vi "Modules Selector.vi"(7 "Scan All":bool, 8 "Module In Dependencies?":bool[](array[boolean]), 10 "Modules Types In":T1[](array[typedef]), 11 "DQMH Modules In":refnum<vi>[](array[refnum])) -> (0 "Module In Dependencies?Out":bool[](array[boolean]), 1 "Descriptions":string[](array[string]), 2 "Modules Types Out":T1[](array[typedef]), 3 "DQMH Modules Out":refnum<vi>[](array[refnum]), 4 "Scan?":bool)   [LabVIEW 2021, in "Panther Dashboard.lvlib"]
uses:
  Panther Dashboard.lvlib
  Module type--enum.ctl
  Module to scan--cluster.ctl
panel:
  in  "DQMH Modules found in Project":T2[](array[typedef])
  in  "Scan Selection":bool
  in  "Select/Unselect All":bool
types:
  T1 = typedef "Panther Dashboard.lvlib/Module type--enum.ctl" = enum16{"Module type: Singleton", "Module type: Cloneable"}
  T2 = typedef "Panther Dashboard.lvlib/Module to scan--cluster.ctl" = cluster{"Module Name":string, "Description":string, "Scan?":bool, "Dependency":bool}
  T3 = enum8{"Enabled", "Disabled", "Disabled and Grayed Out"}
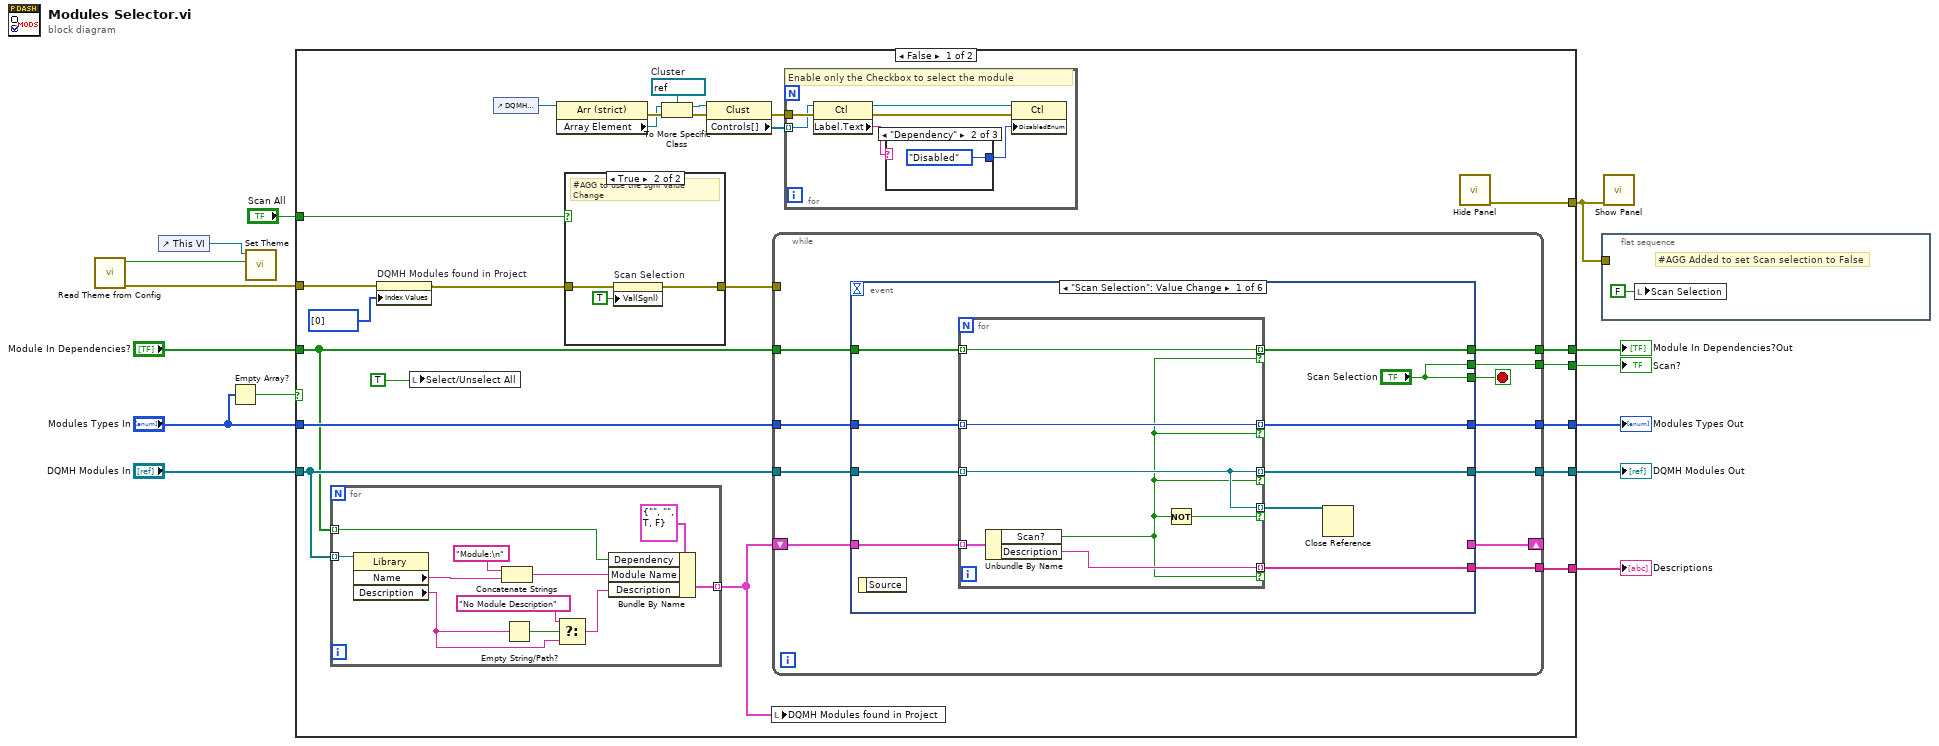
[diagram p0: block diagram]
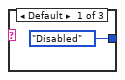
[diagram p3: hidden frame]
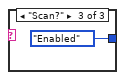
[diagram p4: hidden frame]
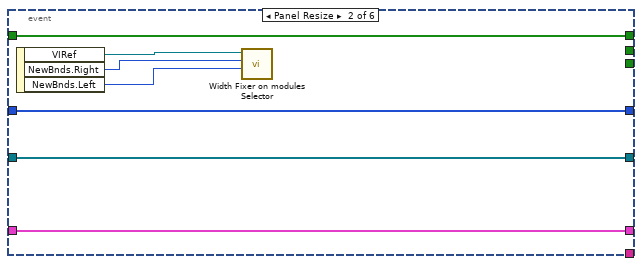
[diagram p5: hidden frame]
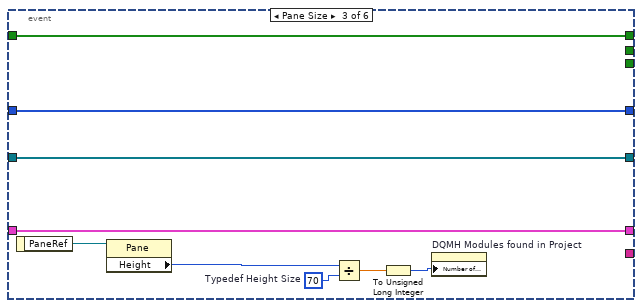
[diagram p6: hidden frame]
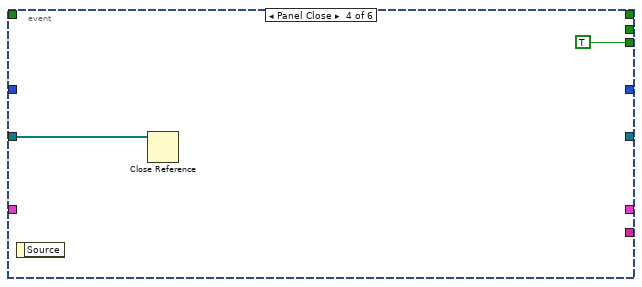
[diagram p7: hidden frame]
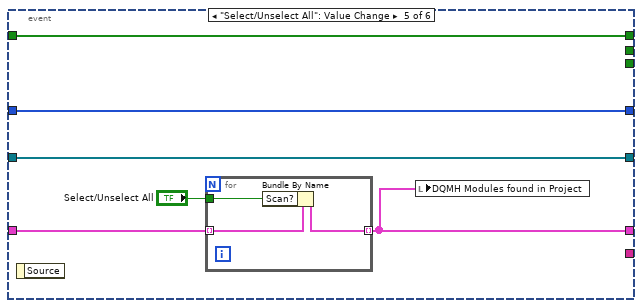
[diagram p8: hidden frame]
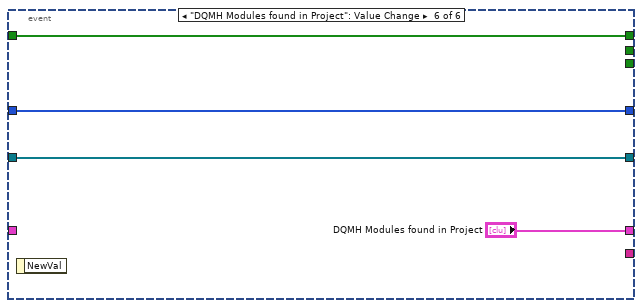
[diagram p9: hidden frame]
diagram:
  n1 = call "Read Theme from Config.vi"() -> ("error out"=w14:errorcluster, "Theme"=w9:bool)  [unwired: 10 in]
  n2 = control-ref of="This VI"() -> (w10:refnum<vi>)
  n3 = Empty Array?(array="Modules Types In") -> (empty?=w7:bool)
  n4 = call "Set Theme.vi"("Dark?"=w9, "VI in"=w10) -> ()  [unwired: 10 in]
  n5 = case shown="False" w7 {
    tunnel: "DQMH Modules In" -> [w29 _]
    tunnel: [w33 _] -> w6
    tunnel: "Modules Types In" -> [w32 _]
    tunnel: [w31 _] -> w12
    tunnel: [w30 _] -> w11
    tunnel: w14 -> [w37 _]
    tunnel: [w38 _] -> w2
    tunnel: "Module In Dependencies?" -> [w24 _]
    tunnel: [w25 _] -> w4
    tunnel: [w18 _] -> w3
    tunnel: "Scan All" -> [w15 _]
    frame False {
      w19 = refnum<vi> refnum  # Cluster
      n6 = for {
        tunnel: w29 -> [w62] mode=indexing
        tunnel: [w61] -> w28 mode=indexing
        tunnel: w24 -> [w52] mode=indexing
        n7 = property class="Library"(reference=w62) -> ("Name"=w59:string, "Description"=w57:string)  [unwired: 1 in, 2 out]
        n8 = Concatenate Strings("Module:\n" ("string"), w59) -> (w54:string)
        n9 = Empty String/Path?(string/path=w57) -> (empty?=w58:bool)
        n10 = Select(t="No Module Description", s=w58, f=w57) -> (s? t:f=w56:string)
        n11 = Bundle By Name(cluster=T2 {"Module Name"="", "Description"="", "Scan?"=TRUE, "Dependency"=FALSE} ("Module"), "Dependency"=w52, "Module Name"=w54, "Description"=w56) -> (w61:T2)
      }
      n12 = property on="DQMH Modules found in Project" class="Arr (strict)"(error in=w37, "Index Values"=u32[] [0]) -> (error out=w16:errorcluster)  [unwired: 1 in, 1 out]
      n13 = local write "Select/Unselect All"(TRUE ("Select /Unselect All Modules")) -> ()
      n14 = control-ref of="DQMH Modules found in Project"() -> (w20:refnum<vi>)
      n15 = property class="Arr (strict)"(reference=w20) -> (error out=w34:errorcluster, "Array Element"=w21:refnum<vi>)  [unwired: 1 in, 1 out]
      n16 = case shown="True" w15 {
        tunnel: [w39 w42] -> w17
        tunnel: w16 -> [w39 w41]
        frame False {
        }
        frame True {
          # "#AGG to use the sgnl Value Change"
          n17 = property on="Scan Selection" class="Bool (strict)"(error in=w41, "Val(Sgnl)"=TRUE ("Value (Signaling)")) -> (error out=w42:errorcluster)  [unwired: 1 in, 1 out]
        }
      }
      n18 = To More Specific Class(target class=w19, reference=w21, error in=w34) -> (specific class reference=w22:refnum<vi>, error out=w35:errorcluster)
      n19 = property class="Clust"(reference=w22, error in=w35) -> (error out=w36:errorcluster, "Controls[]"=w23:refnum<vi>[])  [unwired: 1 out]
      n20 = local write "DQMH Modules found in Project"(w28) -> ()
      n21 = while {
        shift-right: [w72] -> _
        shift-left: w28 -> [w73]
        tunnel: w29 -> [w71]
        tunnel: [w70] -> w33
        tunnel: w32 -> [w69]
        tunnel: [w68] -> w31
        tunnel: [w67] -> w30
        tunnel: w24 -> [w66]
        tunnel: [w65] -> w25
        tunnel: [w63] -> w18
        tunnel: w17 -> [_]
        stop <- w64 stop-if-true
        n22 = event shown="[0] \"Scan Selection\": Value Change" {
          selector: _ -> [_ _ _ _ _ _]
          dyn-events: _ -> [_ _ _ _ _ _]
          timeout: _ -> [_ _ _ _ _ _]
          tunnel: w73 -> [w83 w95 w102 _ w112 _]
          tunnel: ["Scan Selection" _ _ TRUE ("All") _ _] -> w64
          tunnel: [_ w95 w102 _ w111 "DQMH Modules found in Project"] -> w72
          tunnel: [w79 w96 w100 _ w113 w121] -> w70
          tunnel: w71 -> [w81 w96 w100 w107 w113 w121]
          tunnel: w69 -> [w82 w97 w101 _ w114 w120]
          tunnel: [w80 w97 w101 _ w114 w120] -> w68
          tunnel: [w78 _ _ _ _ _] -> w67
          tunnel: w66 -> [w76 w91 w98 _ w109 w118]
          tunnel: [w75 w91 w98 _ w109 w118] -> w65
          tunnel: ["Scan Selection" _ _ _ _ _] -> w63
          event "Scan Selection": Value Change {
            n23 = event-data() -> ()  [unwired: 1 in, 1 out]
            n24 = for {
              tunnel: w83 -> [w90] mode=indexing
              tunnel: [w89] -> w78 mode=indexing if=w84
              tunnel: w82 -> [w88] mode=indexing
              tunnel: w81 -> [w87] mode=indexing
              tunnel: [w88] -> w80 mode=indexing if=w84
              tunnel: [w87] -> w79 mode=indexing if=w84
              tunnel: [w87] -> w77 mode=indexing if=w86
              tunnel: w76 -> [w85] mode=indexing
              tunnel: [w85] -> w75 mode=indexing if=w84
              n25 = Unbundle By Name(w90) -> ("Scan?"=w84:bool, "Description"=w89:string)
              n26 = Not(x=w84) -> (.not. x?=w86:bool)
            }
            n27 = Close Reference(reference=w77) -> ()  [unwired: 1 in, 1 out]
          }
          event Panel Resize {
            n28 = event-data() -> ("VIRef"=w94:refnum<vi>, "NewBnds.Right"=w92:i16, "NewBnds.Left"=w93:i16)  [unwired: 1 in]
            n29 = call "Width Fixer on modules Selector.vi"("Left"=w93, "Right"=w92, "VI in"=w94) -> ()  [unwired: 9 in]
          }
          event Pane Size {
            w104 = u32 70  # Typedef Height Size
            n30 = event-data() -> ("PaneRef"=w106:refnum<vi>)  [unwired: 1 in]
            n31 = property class="Pane"(reference=w106) -> ("Height"=w105:u32)  [unwired: 1 in, 2 out]
            n32 = Divide(x=w105, y=w104) -> (x/y=w103:dbl)
            n33 = To Unsigned Long Integer(number=w103) -> (unsigned 32bit integer=w99:u32)
            n34 = property on="DQMH Modules found in Project" class="Arr (strict)"("Number of Rows"=w99) -> ()  [unwired: 2 in, 2 out]
          }
          event Panel Close {
            n35 = event-data() -> ()  [unwired: 1 in, 1 out]
            n36 = Close Reference(reference=w107) -> ()  [unwired: 1 in, 1 out]
          }
          event "Select/Unselect All": Value Change {
            n37 = event-data() -> ()  [unwired: 1 in, 1 out]
            n38 = for {
              tunnel: w112 -> [w117] mode=indexing
              tunnel: [w116] -> w111 mode=indexing
              tunnel: "Select/Unselect All" -> [w115]
              n39 = Bundle By Name(cluster=w117, "Scan?"=w115) -> (w116:T2)
            }
            n40 = local write "DQMH Modules found in Project"(w111) -> ()
          }
          event "DQMH Modules found in Project": Value Change {
            n41 = event-data() -> ()  [unwired: 1 in, 1 out]
          }
        }
      }
      n42 = for {
        tunnel: w23 -> [w46] mode=indexing
        tunnel: w36 -> [w48]
        # "Enable only the Checkbox to select the module"
        n43 = property class="Ctl"(reference=w46, error in=w48) -> (reference out=w44:refnum<vi>, error out=w47:errorcluster, "Label.Text"=w45:string)
        n44 = case shown="\"Dependency\"" w45 {
          tunnel: [T3."Disabled" ("Disabled") T3."Disabled" ("Disabled") T3."Enabled" ("Disabled")] -> w43
          frame Default {
          }
          frame "Dependency" {
          }
          frame "Scan?" {
          }
        }
        n45 = property class="Ctl"(reference=w44, error in=w47, "DisabledEnum"=w43) -> ()  [unwired: 2 out]
      }
      n46 = call "Hide Panel.vi"() -> ("error out"=w38:errorcluster)  [unwired: 11 in]
    }
    frame True {
    }
  }
  "Modules Types Out" <- w12
  "DQMH Modules Out" <- w6
  "Descriptions" <- w11
  "Module In Dependencies?Out" <- w4
  "Scan?" <- w3
  n47 = flat-sequence {
    tunnel: w2 -> [_]
    frame #0 {
      # "#AGG Added to set Scan selection to False"
      n48 = local write "Scan Selection"(FALSE ("Scan Selection")) -> ()
    }
  }
  n49 = call "Show Panel.vi"("error in (no error)"=w2) -> ()  [unwired: 10 in, 1 out]
